vi "nm.cm-1.vi"(11 "nm or cm-1 in":dbl) -> (3 "cm-1 or nm  out":dbl)   [LabVIEW 2022 SP3]
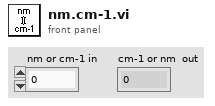
[diagram p1: front panel]
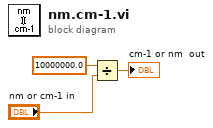
[diagram p0: block diagram]
diagram:
  n1 = Divide(x=10000000.0 ("y"), y="nm or cm-1 in") -> (x/y=→"cm-1 or nm  out":dbl)
